vi "grafico.vi"() -> ()   [LabVIEW 2014]
uses:
  <vilib>/Utility/file.llb/Read From Spreadsheet File (DBL).vi
panel:
  out "VISUALIZAR SINAL":cluster{"all rows":dbl[], "all rows":dbl[]}[](graph)
  in  "CARREGA ARQUIVO":bool
  in  "?":bool
  in  "SLR1":bool
  in  "ST3":bool
  in  "ST2":bool
  in  "ST1":bool
  in  "VDC":bool
  in  "IDC":bool
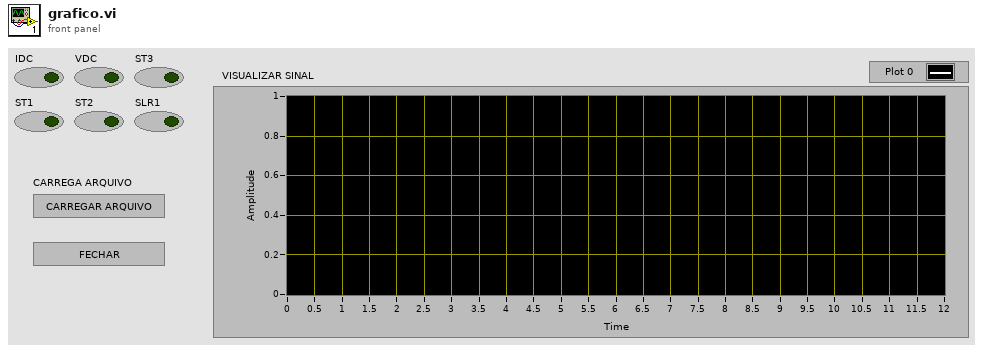
[diagram p1: front panel]
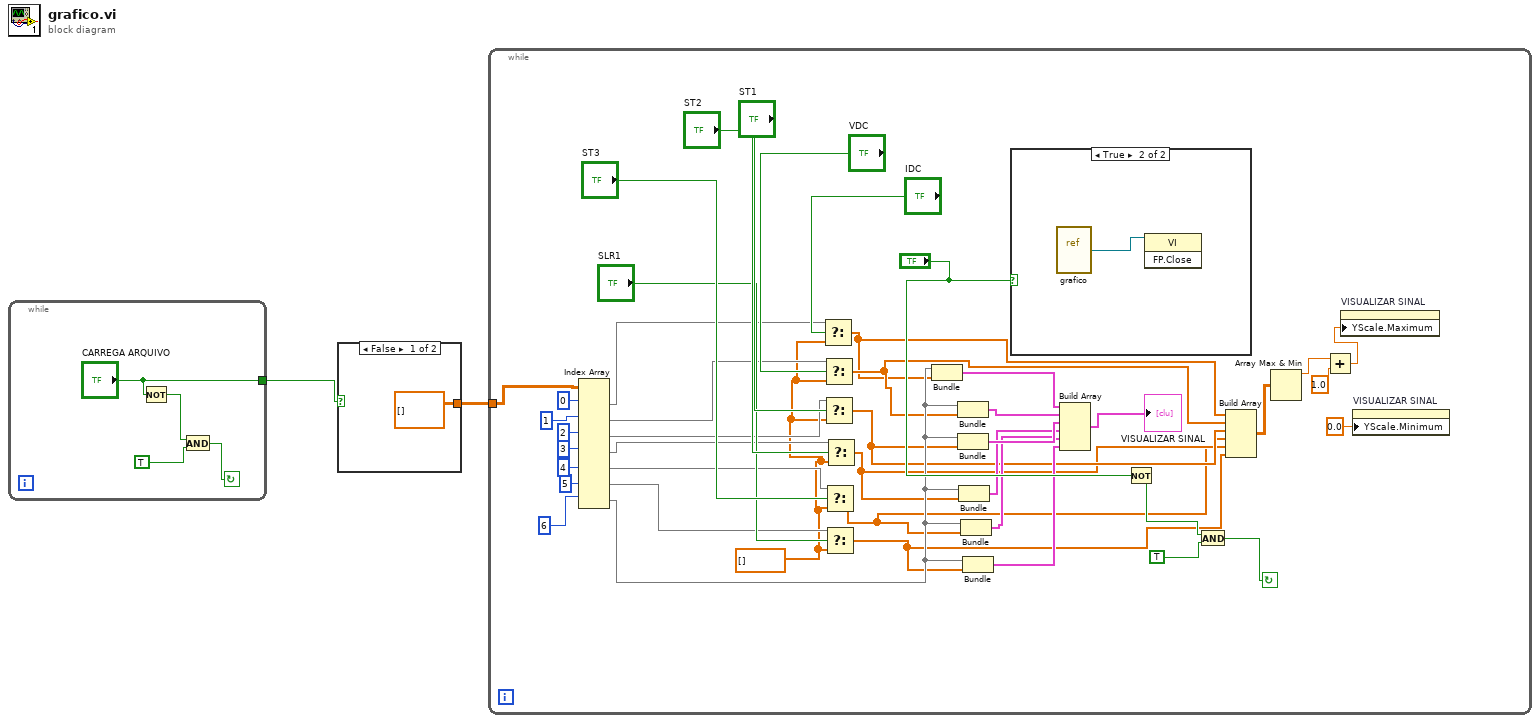
[diagram p0: block diagram]
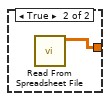
[diagram p2: hidden frame]
diagram:
  n1 = while {
    tunnel: ["CARREGA ARQUIVO"] -> w2
    stop <- w4 continue-if-true
    n2 = Not(x="CARREGA ARQUIVO") -> (.not. x?=w5:bool)
    n3 = And(x=w5, y=TRUE) -> (x .and. y?=w4:bool)
  }
  n4 = case shown="False" w2 {
    tunnel: [dbl[][] [] ("all rows") w8] -> w1
    frame False {
    }
    frame True {
      n5 = call-poly <vilib>:"Read From Spreadsheet File.vi"() -> ("all rows"=w8:dbl[][])  [unwired: 7 in, 4 out]
    }
  }
  n6 = while {
    tunnel: w1 -> [w13]
    stop <- w31 continue-if-true
    w12 = dbl[] [] ("f")
    n7 = Index Array(array=w13, index (row) #1=0 ("index (row)"), index (row) #2=1 ("index (row)"), index (row) #3=2 ("index (row)"), index (row) #4=3 ("index (row)"), index (row) #5=4 ("index (row)"), index (row) #6=5 ("index (row)"), index (row) #7=6 ("index (row)")) -> (element #1=w35:dbl[], element #2=w40:dbl[], element #3=w39:dbl[], element #4=w38:dbl[], element #5=w37:dbl[], element #6=w36:dbl[], element #7=w29:dbl[])  [unwired: 7 in]
    n8 = Select(t=w35, s="IDC", f=w12) -> (s? t:f=w11:dbl[])
    n9 = Select(t=w40, s="VDC", f=w12) -> (s? t:f=w18:dbl[])
    n10 = Select(t=w39, s="ST1", f=w12) -> (s? t:f=w17:dbl[])
    n11 = Select(t=w37, s="ST3", f=w12) -> (s? t:f=w15:dbl[])
    n12 = Select(t=w36, s="SLR1", f=w12) -> (s? t:f=w9:dbl[])
    n13 = Select(t=w38, s="ST2", f=w12) -> (s? t:f=w16:dbl[])
    n14 = Bundle("all rows"=w29, "f"=w11) -> (w28:cluster{"all rows":dbl[], "f":dbl[]})  [unwired: 1 in]
    n15 = Bundle("all rows"=w29, "f"=w18) -> (w27:cluster{"all rows":dbl[], "f":dbl[]})  [unwired: 1 in]
    n16 = Bundle("all rows"=w29, "f"=w17) -> (w26:cluster{"all rows":dbl[], "f":dbl[]})  [unwired: 1 in]
    n17 = Bundle("all rows"=w29, "f"=w16) -> (w25:cluster{"all rows":dbl[], "f":dbl[]})  [unwired: 1 in]
    n18 = Bundle("all rows"=w29, "f"=w15) -> (w24:cluster{"all rows":dbl[], "f":dbl[]})  [unwired: 1 in]
    n19 = Bundle("all rows"=w29, "f"=w9) -> (w23:cluster{"all rows":dbl[], "f":dbl[]})  [unwired: 1 in]
    n20 = case shown="True" "?" {
      frame False {
      }
      frame True {
        n21 = vi-ref "grafico.vi"() -> (w53:refnum<vi>)
        n22 = invoke class="VI" method="FP.Close"(reference=w53) -> ()  [unwired: 2 in, 3 out]
      }
    }
    n23 = Build Array(w28, w27, w26, w25, w24, w23) -> (→"VISUALIZAR SINAL":cluster{"all rows":dbl[], "f":dbl[]}[])
    n24 = Not(x="?") -> (.not. x?=w33:bool)
    n25 = And(x=w33, y=TRUE) -> (x .and. y?=w31:bool)
    n26 = Build Array(w11, w18, w17, w16, w15, w9) -> (w10:dbl[][])
    n27 = Array Max & Min(array=w10) -> (max value=w14:dbl)  [unwired: 3 out]
    n28 = Add(x=w14, y=1.0) -> (x+y=w19:dbl)
    n29 = property on="VISUALIZAR SINAL" class="XYGraph (strict)"("YScale.Maximum"=w19) -> ()  [unwired: 2 in, 2 out]
    n30 = property on="VISUALIZAR SINAL" class="XYGraph (strict)"("YScale.Minimum"=0.0 ("Y Scale.Range:Minimum")) -> ()  [unwired: 2 in, 2 out]
  }
